vi "Lab Panel V5.22.vi"() -> ()   [LabVIEW 2013] (continued)
              n180 = call "sub vi - GET ALL TEMP v7.vi"("LA01-EN"=w224, "simulate"=w186, "LA02-EN"=w224, "LA03-EN"=w224, "LA04-EN"=w224, "LA05-EN"=w224, "Gen Cal Value"=1) -> ("LA01 TEMP"=w222:T24, "LA02 TEMP"=w215:T24, "LA03 TEMP"=w208:T24, "LA04 TEMP"=w201:T24, "LA05 TEMP"=w194:T24)  [unwired: 3 in, 1 out]
              n181 = local write "LAB05 TEMP"(w194) -> ()
              n182 = local write "LAB04 TEMP"(w201) -> ()
              n183 = Unbundle(w208) -> ("T1"=w205:dbl, "T2"=w204:dbl, "T3"=w203:dbl, "T4"=w202:dbl)  [unwired: 2 out]
              n184 = Unbundle(w222) -> ("T1"=w220:dbl, "T2"=w219:dbl, "T3"=w218:dbl, "T4"=w217:dbl)  [unwired: 2 out]
              n185 = Unbundle(w215) -> ("T1"=w212:dbl, "T2"=w211:dbl, "T3"=w210:dbl, "T4"=w209:dbl)  [unwired: 2 out]
              n186 = Unbundle(w201) -> ("T1"=w199:dbl, "T2"=w198:dbl, "T3"=w197:dbl, "T4"=w196:dbl)  [unwired: 2 out]
              n187 = Unbundle(w194) -> ("T1"=w192:dbl, "T2"=w191:dbl, "T3"=w190:dbl, "T4"=w189:dbl)  [unwired: 2 out]
              n188 = local write "LAB01 TEMP"(w222) -> ()
              n189 = local write "LAB02 TEMP"(w215) -> ()
              n190 = local write "LAB03 TEMP"(w208) -> ()
              n191 = local read "TEMP LA05"() -> (w193:T9)
              n192 = local read "TEMP LA04"() -> (w200:T9)
              n193 = local read "TEMP LA02"() -> (w214:T9)
              n194 = local read "TEMP LA03"() -> (w207:T9)
              n195 = local read "TEMP LA01"() -> (w221:T9)
              n196 = Bundle(cluster=w207, "TL-1"=w205, "TN-1"=w204, "TL-2"=w203, "TN-2"=w202) -> (w206:T9)  [unwired: 4 in]
              n197 = Bundle(cluster=w221, "TL-1"=w220, "TN-1"=w219, "TL-2"=w218, "TN-2"=w217) -> (w216:T9)  [unwired: 4 in]
              n198 = Bundle(cluster=w214, "TL-1"=w212, "TN-1"=w211, "TL-2"=w210, "TN-2"=w209) -> (w213:T9)  [unwired: 4 in]
              n199 = Bundle(cluster=w200, "TL-1"=w199, "TN-1"=w198, "TL-2"=w197, "TN-2"=w196) -> (w195:T9)  [unwired: 4 in]
              n200 = Bundle(cluster=w193, "TL-1"=w192, "TN-1"=w191, "TL-2"=w190, "TN-2"=w189) -> (w188:T9)  [unwired: 4 in]
              n201 = local write "TEMP LA03"(w206) -> ()
              n202 = local write "TEMP LA01"(w216) -> ()
              n203 = local write "TEMP LA02"(w213) -> ()
              n204 = local write "TEMP LA05"(w188) -> ()
              n205 = local write "TEMP LA04"(w195) -> ()
            }
            frame #2 {
              w235 = 0
              n206 = local read "LAB01 TEMP"() -> (w237:T12)
              n207 = local read "SIG LAB01-2"() -> (w232:T2)
              n208 = Unbundle By Name(w237) -> ("T1 Live"=w230:dbl, "T1 Neut"=w229:dbl, "T2 Live"=w228:dbl, "T2 Neut"=w227:dbl)  [unwired: 2 out]
              n209 = local read "SIG LAB01-1"() -> (w234:T2)
              n210 = local read "TEMP LA01"() -> (w238:T9)
              n211 = Bundle By Name(cluster=w238, "TL-1"=w230, "TN-1"=w229, "TL-2"=w228, "TN-2"=w227, "TL -1COUNT"=w235, "TN-1 COUNT"=w235, "TL-2 COUNT"=w235, "TN-2 COUNT"=w235) -> (w236:T9)
              n212 = Bundle(cluster=w234, "Tmp Live"=w230, "Tmp Neut"=w229) -> (w233:T2)  [unwired: 3 in]
              n213 = Bundle(cluster=w232, "Tmp Live"=w228, "Tmp Neut"=w227) -> (w231:T2)  [unwired: 3 in]
              n214 = local write "SIG LAB01-2"(w231) -> ()
              n215 = local write "SIG LAB01-1"(w233) -> ()
              n216 = local write "TEMP LA01"(w236) -> ()
            }
            frame #3 {
              w247 = 0
              n217 = local read "LAB02 TEMP"() -> (w249:T12)
              n218 = Unbundle By Name(w249) -> ("T1 Live"=w242:dbl, "T1 Neut"=w241:dbl, "T2 Live"=w240:dbl, "T2 Neut"=w239:dbl)  [unwired: 2 out]
              n219 = local read "SIG LAB02-1"() -> (w246:T2)
              n220 = local read "SIG LAB02-2"() -> (w245:T2)
              n221 = local read "TEMP LA02"() -> (w250:T9)
              n222 = Bundle By Name(cluster=w250, "TL-1"=w242, "TN-1"=w241, "TL-2"=w240, "TN-2"=w239, "TL -1COUNT"=w247, "TN-1 COUNT"=w247, "TL-2 COUNT"=w247, "TN-2 COUNT"=w247) -> (w248:T9)
              n223 = Bundle(cluster=w245, "Tmp Live"=w240, "Tmp Neut"=w239) -> (w243:T2)  [unwired: 3 in]
              n224 = Bundle(cluster=w246, "Tmp Live"=w242, "Tmp Neut"=w241) -> (w244:T2)  [unwired: 3 in]
              n225 = local write "TEMP LA02"(w248) -> ()
              n226 = local write "SIG LAB02-1"(w244) -> ()
              n227 = local write "SIG LAB02-2"(w243) -> ()
            }
            frame #4 {
              w259 = 0
              n228 = local read "LAB03 TEMP"() -> (w261:T12)
              n229 = Unbundle By Name(w261) -> ("T1 Live"=w254:dbl, "T1 Neut"=w253:dbl, "T2 Live"=w252:dbl, "T2 Neut"=w251:dbl)  [unwired: 2 out]
              n230 = local read "SIG LAB03-1"() -> (w258:T2)
              n231 = local read "SIG LAB03-2"() -> (w257:T2)
              n232 = local read "TEMP LA03"() -> (w262:T9)
              n233 = Bundle By Name(cluster=w262, "TL-1"=w254, "TN-1"=w253, "TL-2"=w252, "TN-2"=w251, "TL -1COUNT"=w259, "TN-1 COUNT"=w259, "TL-2 COUNT"=w259, "TN-2 COUNT"=w259) -> (w260:T9)
              n234 = Bundle(cluster=w257, "Tmp Live"=w252, "Tmp Neut"=w251) -> (w255:T2)  [unwired: 3 in]
              n235 = Bundle(cluster=w258, "Tmp Live"=w254, "Tmp Neut"=w253) -> (w256:T2)  [unwired: 3 in]
              n236 = local write "TEMP LA03"(w260) -> ()
              n237 = local write "SIG LAB03-2"(w255) -> ()
              n238 = local write "SIG LAB03-1"(w256) -> ()
            }
            frame #5 {
              w271 = 0
              n239 = local read "LAB04 TEMP"() -> (w273:T12)
              n240 = Unbundle By Name(w273) -> ("T1 Live"=w266:dbl, "T1 Neut"=w265:dbl, "T2 Live"=w264:dbl, "T2 Neut"=w263:dbl)  [unwired: 2 out]
              n241 = local read "SIG LAB04-2"() -> (w269:T2)
              n242 = local read "SIG LAB04-1"() -> (w270:T2)
              n243 = local read "TEMP LA04"() -> (w274:T9)
              n244 = Bundle By Name(cluster=w274, "TL-1"=w266, "TN-1"=w265, "TL-2"=w264, "TN-2"=w263, "TL -1COUNT"=w271, "TN-1 COUNT"=w271, "TL-2 COUNT"=w271, "TN-2 COUNT"=w271) -> (w272:T9)
              n245 = Bundle(cluster=w269, "Tmp Live"=w264, "Tmp Neut"=w263) -> (w267:T2)  [unwired: 3 in]
              n246 = Bundle(cluster=w270, "Tmp Live"=w266, "Tmp Neut"=w265) -> (w268:T2)  [unwired: 3 in]
              n247 = local write "SIG LAB04-2"(w267) -> ()
              n248 = local write "TEMP LA04"(w272) -> ()
              n249 = local write "SIG LAB04-1"(w268) -> ()
            }
            frame #6 {
              w283 = 0
              n250 = local read "LAB05 TEMP"() -> (w285:T12)
              n251 = Unbundle By Name(w285) -> ("T1 Live"=w278:dbl, "T1 Neut"=w277:dbl, "T2 Live"=w276:dbl, "T2 Neut"=w275:dbl)  [unwired: 2 out]
              n252 = local read "SIG LAB05-2"() -> (w281:T2)
              n253 = local read "SIG LAB05-1"() -> (w282:T2)
              n254 = local read "TEMP LA05"() -> (w286:T9)
              n255 = Bundle By Name(cluster=w286, "TL-1"=w278, "TN-1"=w277, "TL-2"=w276, "TN-2"=w275, "TL -1COUNT"=w283, "TN-1 COUNT"=w283, "TL-2 COUNT"=w283, "TN-2 COUNT"=w283) -> (w284:T9)
              n256 = Bundle(cluster=w281, "Tmp Live"=w276, "Tmp Neut"=w275) -> (w279:T2)  [unwired: 3 in]
              n257 = Bundle(cluster=w282, "Tmp Live"=w278, "Tmp Neut"=w277) -> (w280:T2)  [unwired: 3 in]
              n258 = local write "SIG LAB05-2"(w279) -> ()
              n259 = local write "SIG LAB05-1"(w280) -> ()
              n260 = local write "TEMP LA05"(w284) -> ()
            }
          }
        }
        frame #8 {
          # "enable front panel, all settings done"
          n261 = property on="Tab Control 2" class="TabCtl (strict)"("DisabledEnum"=T16."Enabled" ("Disabled")) -> ()  [unwired: 2 in, 2 out]
          n262 = property on="Tab Control 2" class="TabCtl (strict)"("Value"=0) -> ()  [unwired: 2 in, 2 out]
        }
        frame #9 {
          n263 = property on="Tab Control 2" class="TabCtl (strict)"("Value"=0) -> ()  [unwired: 2 in, 2 out]
        }
      }
    }
    frame #2 {
      n264 = node-c288("loop  delay(mS)") -> (w292:T17)  [unwired: 3 in]
      n265 = timed-loop {
        timing: w292 -> [_]
        timing-out: [_] -> w291
        i -> [w318]
        stop <- w294 stop-if-true
        n266 = node-c288() -> ()  [unwired: 1 in, 1 out]
        n267 = local read "Resets Done"() -> (w297:dbl)
        n268 = Greater?(x=w297, y=10) -> (0:w293:bool)
        n269 = local read "SELECT LAB05-2"() -> (w298:T3)
        n270 = local read "SELECT LAB05-1"() -> (w299:T3)
        n271 = local read "SELECT LAB04-2"() -> (w300:T3)
        n272 = local read "SELECT LAB03-1"() -> (w303:T3)
        n273 = local read "SELECT LAB02-2"() -> (w304:T3)
        n274 = local read "SELECT LAB01-1"() -> (w307:T3)
        n275 = local read "SELECT LAB03-2"() -> (w302:T3)
        n276 = local read "SELECT LAB01-2"() -> (w306:T3)
        n277 = local read "SELECT LAB04-1"() -> (w301:T3)
        n278 = Or(x=w293, y="stop") -> (x .or. y?=w294:bool)
        n279 = local read "SELECT LAB02-1"() -> (w305:T3)
        n280 = local read "run lab03-2"() -> (w312:bool)
        n281 = local read "run lab04-1"() -> (w311:bool)
        n282 = local read "run lab05-1"() -> (w309:bool)
        n283 = local read "run lab04-2"() -> (w310:bool)
        n284 = local read "run lab05-2"() -> (w308:bool)
        n285 = local read "run lab03-1"() -> (w313:bool)
        n286 = local read "run lab02-2"() -> (w314:bool)
        n287 = local read "run lab02-1"() -> (w315:bool)
        n288 = local read "run lab01-1"() -> (w317:bool)
        n289 = local read "run lab01-2"() -> (w316:bool)
        n290 = global write "Global display 1.vi" "stop disp"(w294) -> ()
        n291 = stacked-sequence {
          seq-local: [_ w384 _ _ _ _ _ _ _ _ _ _ _ _ _ _ _ _ _ _ _ _ _] -> [_ _ _ _ _ w2485 _ _ _ _ _ _ _ _ _ _ _ _ _ _ _ _ _]
          seq-local: [_ w383 _ _ _ _ _ _ _ _ _ _ _ _ _ _ _ _ _ _ _ _ _] -> [_ _ _ _ _ w2484 _ _ _ _ _ _ _ _ _ _ _ _ _ _ _ _ _]
          seq-local: [_ w370 _ _ _ _ _ _ _ _ _ _ _ _ _ _ _ _ _ _ _ _ _] -> [_ _ _ _ _ w2483 _ _ _ _ _ _ _ _ _ _ _ _ _ _ _ _ _]
          seq-local: [_ w369 _ _ _ _ _ _ _ _ _ _ _ _ _ _ _ _ _ _ _ _ _] -> [_ _ _ _ _ w2482 _ _ _ _ _ _ _ _ _ _ _ _ _ _ _ _ _]
          seq-local: [_ w368 _ _ _ _ _ _ _ _ _ _ _ _ _ _ _ _ _ _ _ _ _] -> [_ _ _ _ _ w2481 _ _ _ _ _ _ _ _ _ _ _ _ _ _ _ _ _]
          seq-local: [_ w367 _ _ _ _ _ _ _ _ _ _ _ _ _ _ _ _ _ _ _ _ _] -> [_ _ _ _ _ w2480 _ _ _ _ _ _ _ _ _ _ _ _ _ _ _ _ _]
          seq-local: [_ w366 _ _ _ _ _ _ _ _ _ _ _ _ _ _ _ _ _ _ _ _ _] -> [_ _ _ _ _ w2479 _ _ _ _ _ _ _ _ _ _ _ _ _ _ _ _ _]
          seq-local: [_ w365 _ _ _ _ _ _ _ _ _ _ _ _ _ _ _ _ _ _ _ _ _] -> [_ _ _ _ _ w2478 _ _ _ _ _ _ _ _ _ _ _ _ _ _ _ _ _]
          seq-local: [_ w364 _ _ _ _ _ _ _ _ _ _ _ _ _ _ _ _ _ _ _ _ _] -> [_ _ _ _ _ w2477 _ _ _ _ _ _ _ _ _ _ _ _ _ _ _ _ _]
          seq-local: [_ w363 _ _ _ _ _ _ _ _ _ _ _ _ _ _ _ _ _ _ _ _ _] -> [_ _ _ _ _ w2476 _ _ _ _ _ _ _ _ _ _ _ _ _ _ _ _ _]
          tunnel: w317 -> [_ _ w400 w648 w2075 w2505 w2820 w3307 _ _ _ _ w3867 _ w4824 _ _ w5112 w5415 w5597 _ _ _]
          tunnel: w316 -> [_ _ w399 w646 w2074 w2504 w2821 w3306 _ _ _ _ w3866 _ w4822 _ _ w5111 w5414 w5595 _ _ _]
          tunnel: w315 -> [_ _ w398 w644 w2073 w2503 w2819 w3305 _ _ _ _ w3865 _ w4820 _ _ w5110 w5413 w5594 _ _ _]
          tunnel: w314 -> [_ _ w397 w642 w2072 w2502 w2818 w3304 _ _ _ _ w3864 _ w4818 _ _ w5109 w5412 w5593 _ _ _]
          tunnel: w313 -> [_ _ w396 w640 w2071 w2501 w2817 w3303 _ _ _ _ w3863 _ w4816 _ _ w5108 w5411 w5592 _ _ _]
          tunnel: w312 -> [_ _ w395 w638 w2070 w2500 w2816 w3302 _ _ _ _ w3862 _ w4814 _ _ w5107 w5410 w5591 _ _ _]
          tunnel: w311 -> [_ _ w394 w636 w2069 w2499 w2815 w3301 _ _ _ _ w3861 _ w4812 _ _ w5106 w5409 w5590 _ _ _]
          tunnel: w310 -> [_ _ w393 w634 w2068 w2498 w2814 w3300 _ _ _ _ w3860 _ w4810 _ _ w5105 w5408 w5589 _ _ _]
          tunnel: w309 -> [_ _ w392 w632 w2067 w2497 w2813 w3299 _ _ _ _ w3859 _ w4808 _ _ w5104 w5407 w5588 _ _ _]
          tunnel: w308 -> [_ _ w391 w630 w2066 w2496 w2812 w3298 _ _ _ _ w3858 _ w4806 _ _ w5103 w5406 w5587 _ _ _]
          tunnel: w307 -> [_ _ _ w647 w2065 w2495 _ _ _ _ _ _ _ _ w4826 _ _ _ _ _ w5942 _ _]
          tunnel: w306 -> [_ _ _ w645 w2064 w2494 _ _ _ _ _ _ _ _ w4821 _ _ _ _ _ w5941 _ _]
          tunnel: w305 -> [_ _ _ w643 w2063 w2493 _ _ _ _ _ _ _ _ w4819 _ _ _ _ _ w5940 _ _]
          tunnel: w304 -> [_ _ _ w641 w2062 w2492 _ _ _ _ _ _ _ _ w4817 _ _ _ _ _ w5939 _ _]
          tunnel: w303 -> [_ _ _ w639 w2061 w2491 _ _ _ _ _ _ _ _ w4815 _ _ _ _ _ w5938 _ _]
          tunnel: w302 -> [_ _ _ w637 w2060 w2490 _ _ _ _ _ _ _ _ w4813 _ _ _ _ _ w5937 _ _]
          tunnel: w301 -> [_ _ _ w635 w2059 w2489 _ _ _ _ _ _ _ _ w4811 _ _ _ _ _ w5936 _ _]
          tunnel: w300 -> [_ _ _ w633 w2058 w2488 _ _ _ _ _ _ _ _ w4809 _ _ _ _ _ w5935 _ _]
          tunnel: w299 -> [_ _ _ w631 w2057 w2487 _ _ _ _ _ _ _ _ w4807 _ _ _ _ _ w5934 _ _]
          tunnel: w298 -> [_ _ _ w629 w2056 w2486 _ _ _ _ _ _ _ _ w4805 _ _ _ _ _ w5933 _ _]
          tunnel: w293 -> [_ _ _ _ _ _ _ _ _ _ _ _ _ _ _ _ _ _ _ _ _ _ w5994]
          frame #0 {
            w326 = FALSE
            w331 = 0.5
            # "set up cycle control"
            n292 = local read "jig cycle"() -> (w330:dbl)
            n293 = local read "Amps Fail level"() -> (w324:dbl)
            n294 = local read "Simulate"() -> (w321:bool)
            n295 = Divide(x="JIG ON TIME (S)", y=w331) -> (x/y=→"on loops":dbl)
            n296 = Divide(x="JIG OFF TIME (S)", y=w331) -> (x/y=→"off loops":dbl)
            n297 = Increment(x=w330) -> (x+1=w329:dbl)
            n298 = local write "Simulate IND"(w321) -> ()
            n299 = global write "Global display 3.vi" "Amps Fail"(w324) -> ()
            n300 = local write "TEMP"(w326) -> ()
            n301 = local write "AI"(w326) -> ()
            n302 = local read "Network Directory"() -> (w323:path)
            n303 = local write "jig cycle"(w329) -> ()
            n304 = call "sub vi - check network dir v2.vi"("PATH"=w323) -> ("error"=w322:bool)  [unwired: 10 in]
            n305 = local write "network error"(w322) -> ()
            n306 = global write "Global display 3.vi" "network drive"(w322) -> ()
            n307 = event shown="[1] \"ADMIN\": Value Change" {
              selector: _ -> [_ _]
              dyn-events: _ -> [_ _]
              timeout: 10 -> [_ _]
              event Timeout {
                n308 = event-data() -> ()  [unwired: 1 in, 3 out]
              }
              event "ADMIN": Value Change {
                n309 = event-data() -> ()  [unwired: 1 in, 6 out]
                n310 = stacked-sequence {
                  seq-local: [_ w335 _] -> [_ _ w336]
                  frame #0 {
                    n311 = global write "Global 1.vi" "password"("9949") -> ()
                  }
                  frame #1 {
                    n312 = call "sub vi - password 1.vi"() -> ("RESULT"=w335:bool)  [unwired: 11 in]
                  }
                  frame #2 {
                    w338 = FALSE
                    n313 = property on="Tab Control 2" class="TabCtl (strict)"() -> ("Pages"=w342:refnum<vi>[])  [unwired: 2 in, 2 out]
                    n314 = Select(t=TRUE, s=w336, f=w338) -> (s? t:f=w337:bool)
                    n315 = Index Array(array=w342, index=8) -> (element=w340:refnum<vi>)
                    n316 = property class="Page"(reference=w340, "PageVis"=w337) -> ()  [unwired: 1 in, 2 out]
                    n317 = local write "ADMIN"(w338) -> ()
                  }
                }
              }
            }
          }
          frame #1 {
            w380 = 60.0
            # "convert temperature rise minutes to cycles"
            n318 = local read "SET LAB05-2"() -> (w344:T5)
            n319 = local read "SET LAB05-1"() -> (w346:T5)
            n320 = local read "SET LAB04-2"() -> (w348:T5)
            n321 = local read "SET LAB01-1"() -> (w362:T5)
            n322 = local read "SET LAB01-2"() -> (w360:T5)
            n323 = local read "SET LAB02-2"() -> (w356:T5)
            n324 = local read "SET LAB04-1"() -> (w350:T5)
            n325 = local read "SET LAB03-1"() -> (w354:T5)
            n326 = local read "SET LAB03-2"() -> (w352:T5)
            n327 = local read "SET LAB02-1"() -> (w358:T5)
            n328 = local read "JIG OFF TIME (S)"() -> (w385:dbl)
            n329 = local read "JIG ON TIME (S)"() -> (w386:dbl)
            n330 = Unbundle(w344) -> ("T-RISE mins"=w343:dbl)  [unwired: 4 out]
            n331 = Unbundle(w346) -> ("T-RISE mins"=w345:dbl)  [unwired: 4 out]
            n332 = Unbundle(w362) -> ("T-RISE mins"=w361:dbl)  [unwired: 4 out]
            n333 = Unbundle(w348) -> ("T-RISE mins"=w347:dbl)  [unwired: 4 out]
            n334 = Unbundle(w360) -> ("T-RISE mins"=w359:dbl)  [unwired: 4 out]
            n335 = Unbundle(w358) -> ("T-RISE mins"=w357:dbl)  [unwired: 4 out]
            n336 = Unbundle(w350) -> ("T-RISE mins"=w349:dbl)  [unwired: 4 out]
            n337 = Unbundle(w356) -> ("T-RISE mins"=w355:dbl)  [unwired: 4 out]
            n338 = Unbundle(w352) -> ("T-RISE mins"=w351:dbl)  [unwired: 4 out]
            n339 = Unbundle(w354) -> ("T-RISE mins"=w353:dbl)  [unwired: 4 out]
            n340 = Add(x=w386, y=w385) -> (x+y=w379:dbl)
            n341 = Multiply(x=w380, y=w351) -> (x*y=w375:dbl)
            n342 = Multiply(x=w380, y=w349) -> (x*y=w374:dbl)
            n343 = Multiply(x=w380, y=w347) -> (x*y=w373:dbl)
            n344 = Multiply(x=w380, y=w345) -> (x*y=w372:dbl)
            n345 = Multiply(x=w380, y=w343) -> (x*y=w371:dbl)
            n346 = Multiply(x=w380, y=w359) -> (x*y=w381:dbl)
            n347 = Multiply(x=w380, y=w353) -> (x*y=w376:dbl)
            n348 = Multiply(x=w380, y=w361) -> (x*y=w382:dbl)
            n349 = Multiply(x=w380, y=w357) -> (x*y=w378:dbl)
            n350 = Multiply(x=w380, y=w355) -> (x*y=w377:dbl)
            n351 = Divide(x=w372, y=w379) -> (x/y=w364:dbl)
            n352 = Divide(x=w373, y=w379) -> (x/y=w365:dbl)
            n353 = Divide(x=w374, y=w379) -> (x/y=w366:dbl)
            n354 = Divide(x=w371, y=w379) -> (x/y=w363:dbl)
            n355 = Divide(x=w376, y=w379) -> (x/y=w368:dbl)
            n356 = Divide(x=w382, y=w379) -> (x/y=w384:dbl)
            n357 = Divide(x=w381, y=w379) -> (x/y=w383:dbl)
            n358 = Divide(x=w378, y=w379) -> (x/y=w370:dbl)
            n359 = Divide(x=w377, y=w379) -> (x/y=w369:dbl)
            n360 = Divide(x=w375, y=w379) -> (x/y=w367:dbl)
          }
          frame #2 {
            # "control cycle loops"
            n361 = local read "JIG OFF TIME (S)"() -> (w389:dbl)
            n362 = local read "JIG ON TIME (S)"() -> (w388:dbl)
            n363 = local read "jig cycle"() -> (w402:dbl)
            n364 = local read "on loops"() -> (w404:dbl)
            n365 = local read "off loops"() -> (w403:dbl)
            n366 = Add(x=w389, y=w388) -> (x+y=w387:dbl)
            n367 = Add(x=w404, y=w403) -> (x+y=w390:dbl)
            n368 = Greater Or Equal?(x=w402, y=w390) -> (x >= y?=w401:bool)
            n369 = case shown="True" w401 {
              tunnel: w400 -> [_ w438]
              tunnel: w399 -> [_ w437]
              tunnel: w398 -> [_ w436]
              tunnel: w397 -> [_ w435]
              tunnel: w396 -> [_ w434]
              tunnel: w395 -> [_ w433]
              tunnel: w394 -> [_ w432]
              tunnel: w393 -> [_ w431]
              tunnel: w392 -> [_ w430]
              tunnel: w391 -> [_ w429]
              tunnel: w387 -> [_ w428]
              frame False {
              }
              frame True {
                # "increment cycle value and convert cycles to minutes for temp rise"
                n370 = stacked-sequence {
                  frame #0 {
                    n371 = local read "Panel #"() -> (w441:dbl)
                    n372 = Increment(x=w441) -> (x+1=w440:dbl)
                    n373 = local write "Panel #"(w440) -> ()
                  }
                  frame #1 {
                    n374 = local read "Panel #"() -> (w442:dbl)
                    n375 = Greater?(x=w442, y=5) -> (0:w444:bool)
                    n376 = case shown="True" w444 {
                      frame False {
                      }
                      frame True {
                        n377 = local write "Panel #"(1) -> ()
                      }
                    }
                  }
                }
                n378 = local read "JIG RELAY CYCLES"() -> (w427:T8)
                n379 = local read "Panel #"() -> (→"Tp Ut":dbl)
                n380 = Unbundle By Name(w427) -> ("LAB01-1"=w425:dbl, "LAB01-2"=w423:dbl, "LAB02-1"=w421:dbl, "LAB02-2"=w419:dbl, "LAB03-1"=w417:dbl, "LAB03-2"=w415:dbl, "LAB04-1"=w413:dbl, "LAB04-2"=w411:dbl, "LAB05-1"=w409:dbl, "LAB05-2"=w407:dbl)
                n381 = stacked-sequence {
                  tunnel: w438 -> [w456 _ _ _ _ _ _ _ _ _]
                  tunnel: w437 -> [_ w473 _ _ _ _ _ _ _ _]
                  tunnel: w436 -> [_ _ w490 _ _ _ _ _ _ _]
                  tunnel: w435 -> [_ _ _ w507 _ _ _ _ _ _]
                  tunnel: w434 -> [_ _ _ _ w524 _ _ _ _ _]
                  tunnel: w433 -> [_ _ _ _ _ w541 _ _ _ _]
                  tunnel: w432 -> [_ _ _ _ _ _ w558 _ _ _]
                  tunnel: w431 -> [_ _ _ _ _ _ _ w575 _ _]
                  tunnel: w430 -> [_ _ _ _ _ _ _ _ w592 _]
                  tunnel: w429 -> [_ _ _ _ _ _ _ _ _ w609]
                  tunnel: w428 -> [w453 w470 w487 w504 w521 w538 w555 w572 w589 w606]
                  tunnel: w425 -> [w447 _ _ _ _ _ _ _ _ _]
                  tunnel: [w446 _ _ _ _ _ _ _ _ _] -> w424
                  tunnel: w423 -> [_ w464 _ _ _ _ _ _ _ _]
                  tunnel: [_ w463 _ _ _ _ _ _ _ _] -> w422
                  tunnel: w421 -> [_ _ w481 _ _ _ _ _ _ _]
                  tunnel: [_ _ w480 _ _ _ _ _ _ _] -> w420
                  tunnel: w419 -> [_ _ _ w498 _ _ _ _ _ _]
                  tunnel: [_ _ _ w497 _ _ _ _ _ _] -> w418
                  tunnel: w417 -> [_ _ _ _ w515 _ _ _ _ _]
                  tunnel: [_ _ _ _ w514 _ _ _ _ _] -> w416
                  tunnel: w415 -> [_ _ _ _ _ w532 _ _ _ _]
                  tunnel: [_ _ _ _ _ w531 _ _ _ _] -> w414
                  tunnel: w413 -> [_ _ _ _ _ _ w549 _ _ _]
                  tunnel: [_ _ _ _ _ _ w548 _ _ _] -> w412
                  tunnel: w411 -> [_ _ _ _ _ _ _ w566 _ _]
                  tunnel: [_ _ _ _ _ _ _ w565 _ _] -> w410
                  tunnel: w409 -> [_ _ _ _ _ _ _ _ w583 _]
                  tunnel: [_ _ _ _ _ _ _ _ w582 _] -> w408
                  tunnel: w407 -> [_ _ _ _ _ _ _ _ _ w600]
                  tunnel: [_ _ _ _ _ _ _ _ _ w599] -> w406
                  frame #0 {
                    n382 = local read "DISP LAB01-1"() -> (w451:T4)
                    n383 = Unbundle(w451) -> ("CYCLE"=w452:dbl)  [unwired: 2 out]
                    n384 = case shown="True" w456 {
                      tunnel: w452 -> [w458 w462]
                      tunnel: [w458 w461] -> w450
                      tunnel: w447 -> [w457 w460]
                      tunnel: [w457 w459] -> w446
                      frame False {
                      }
                      frame True {
                        n385 = Increment(x=w460) -> (x+1=w459:dbl)
                        n386 = Increment(x=w462) -> (x+1=w461:dbl)
                      }
                    }
                    n387 = Multiply(x=w450, y=w453) -> (x*y=w454:dbl)
                    n388 = Divide(x=w454, y=60.0) -> (x/y=w449:dbl)
                    n389 = Bundle(cluster=w451, "CYCLE"=w450, "MINS"=w449) -> (w448:T4)  [unwired: 1 in]
                    n390 = local write "DISP LAB01-1"(w448) -> ()
                  }
                  frame #1 {
                    n391 = local read "DISP LAB01-2"() -> (w468:T4)
                    n392 = Unbundle(w468) -> ("CYCLE"=w469:dbl)  [unwired: 2 out]
                    n393 = case shown="True" w473 {
                      tunnel: w469 -> [w475 w479]
                      tunnel: [w475 w478] -> w466
                      tunnel: w464 -> [w474 w477]
                      tunnel: [w474 w476] -> w463
                      frame False {
                      }
                      frame True {
                        n394 = Increment(x=w477) -> (x+1=w476:dbl)
                        n395 = Increment(x=w479) -> (x+1=w478:dbl)
                      }
                    }
                    n396 = Multiply(x=w466, y=w470) -> (x*y=w471:dbl)
                    n397 = Divide(x=w471, y=60.0) -> (x/y=w465:dbl)
                    n398 = Bundle(cluster=w468, "CYCLE"=w466, "MINS"=w465) -> (w467:T4)  [unwired: 1 in]
                    n399 = local write "DISP LAB01-2"(w467) -> ()
                  }
                  frame #2 {
                    n400 = local read "DISP LAB02-1"() -> (w485:T4)
                    n401 = Unbundle(w485) -> ("CYCLE"=w486:dbl)  [unwired: 2 out]
                    n402 = case shown="True" w490 {
                      tunnel: [w492 w496] -> w483
                      tunnel: w486 -> [w492 w495]
                      tunnel: w481 -> [w491 w494]
                      tunnel: [w491 w493] -> w480
                      frame False {
                      }
                      frame True {
                        n403 = Increment(x=w494) -> (x+1=w493:dbl)
                        n404 = Increment(x=w495) -> (x+1=w496:dbl)
                      }
                    }
                    n405 = Multiply(x=w483, y=w487) -> (x*y=w488:dbl)
                    n406 = Divide(x=w488, y=60.0) -> (x/y=w482:dbl)
                    n407 = Bundle(cluster=w485, "CYCLE"=w483, "MINS"=w482) -> (w484:T4)  [unwired: 1 in]
                    n408 = local write "DISP LAB02-1"(w484) -> ()
                  }
                  frame #3 {
                    n409 = local read "DISP LAB02-2"() -> (w502:T4)
                    n410 = Unbundle(w502) -> ("CYCLE"=w503:dbl)  [unwired: 2 out]
                    n411 = case shown="True" w507 {
                      tunnel: [w509 w513] -> w501
                      tunnel: w503 -> [w509 w512]
                      tunnel: w498 -> [w508 w511]
                      tunnel: [w508 w510] -> w497
                      frame False {
                      }
                      frame True {
                        n412 = Increment(x=w511) -> (x+1=w510:dbl)
                        n413 = Increment(x=w512) -> (x+1=w513:dbl)
                      }
                    }
                    n414 = Multiply(x=w501, y=w504) -> (x*y=w505:dbl)
                    n415 = Divide(x=w505, y=60.0) -> (x/y=w500:dbl)
                    n416 = Bundle(cluster=w502, "CYCLE"=w501, "MINS"=w500) -> (w499:T4)  [unwired: 1 in]
                    n417 = local write "DISP LAB02-2"(w499) -> ()
                  }
                  frame #4 {
                    n418 = local read "DISP LAB03-1"() -> (w519:T4)
                    n419 = Unbundle(w519) -> ("CYCLE"=w520:dbl)  [unwired: 2 out]
                    n420 = case shown="True" w524 {
                      tunnel: [w526 w530] -> w516
                      tunnel: w520 -> [w526 w529]
                      tunnel: w515 -> [w525 w528]
                      tunnel: [w525 w527] -> w514
                      frame False {
                      }
                      frame True {
                        n421 = Increment(x=w528) -> (x+1=w527:dbl)
                        n422 = Increment(x=w529) -> (x+1=w530:dbl)
                      }
                    }
                    n423 = Multiply(x=w516, y=w521) -> (x*y=w522:dbl)
                    n424 = Divide(x=w522, y=60.0) -> (x/y=w517:dbl)
                    n425 = Bundle(cluster=w519, "CYCLE"=w516, "MINS"=w517) -> (w518:T4)  [unwired: 1 in]
                    n426 = local write "DISP LAB03-1"(w518) -> ()
                  }
                  frame #5 {
                    n427 = local read "DISP LAB03-2"() -> (w536:T4)
                    n428 = Unbundle(w536) -> ("CYCLE"=w537:dbl)  [unwired: 2 out]
                    n429 = case shown="True" w541 {
                      tunnel: [w543 w547] -> w535
                      tunnel: w537 -> [w543 w546]
                      tunnel: w532 -> [w542 w545]
                      tunnel: [w542 w544] -> w531
                      frame False {
                      }
                      frame True {
                        n430 = Increment(x=w545) -> (x+1=w544:dbl)
                        n431 = Increment(x=w546) -> (x+1=w547:dbl)
                      }
                    }
                    n432 = Multiply(x=w535, y=w538) -> (x*y=w539:dbl)
                    n433 = Divide(x=w539, y=60.0) -> (x/y=w534:dbl)
                    n434 = Bundle(cluster=w536, "CYCLE"=w535, "MINS"=w534) -> (w533:T4)  [unwired: 1 in]
                    n435 = local write "DISP LAB03-2"(w533) -> ()
                  }
                  frame #6 {
                    n436 = local read "DISP LAB04-1"() -> (w553:T4)
                    n437 = Unbundle(w553) -> ("CYCLE"=w554:dbl)  [unwired: 2 out]
                    n438 = case shown="True" w558 {
                      tunnel: [w560 w564] -> w551
                      tunnel: w554 -> [w560 w563]
                      tunnel: w549 -> [w559 w562]
                      tunnel: [w559 w561] -> w548
                      frame False {
                      }
                      frame True {
                        n439 = Increment(x=w562) -> (x+1=w561:dbl)
                        n440 = Increment(x=w563) -> (x+1=w564:dbl)
                      }
                    }
                    n441 = Multiply(x=w551, y=w555) -> (x*y=w556:dbl)
                    n442 = Divide(x=w556, y=60.0) -> (x/y=w550:dbl)
                    n443 = Bundle(cluster=w553, "CYCLE"=w551, "MINS"=w550) -> (w552:T4)  [unwired: 1 in]
                    n444 = local write "DISP LAB04-1"(w552) -> ()
                  }
                  frame #7 {
                    n445 = local read "DISP LAB04-2"() -> (w570:T4)
                    n446 = Unbundle(w570) -> ("CYCLE"=w571:dbl)  [unwired: 2 out]
                    n447 = case shown="True" w575 {
                      tunnel: [w577 w581] -> w568
                      tunnel: w571 -> [w577 w580]
                      tunnel: w566 -> [w576 w579]
                      tunnel: [w576 w578] -> w565
                      frame False {
                      }
                      frame True {
                        n448 = Increment(x=w579) -> (x+1=w578:dbl)
                        n449 = Increment(x=w580) -> (x+1=w581:dbl)
                      }
                    }
                    n450 = Multiply(x=w568, y=w572) -> (x*y=w574:dbl)
                    n451 = Divide(x=w574, y=60.0) -> (x/y=w567:dbl)
                    n452 = Bundle(cluster=w570, "CYCLE"=w568, "MINS"=w567) -> (w569:T4)  [unwired: 1 in]
                    n453 = local write "DISP LAB04-2"(w569) -> ()
                  }
                  frame #8 {
                    n454 = local read "DISP LAB05-1"() -> (w587:T4)
                    n455 = Unbundle(w587) -> ("CYCLE"=w588:dbl)  [unwired: 2 out]
                    n456 = case shown="True" w592 {
                      tunnel: [w594 w598] -> w585
                      tunnel: w588 -> [w594 w597]
                      tunnel: w583 -> [w593 w596]
                      tunnel: [w593 w595] -> w582
                      frame False {
                      }
                      frame True {
                        n457 = Increment(x=w596) -> (x+1=w595:dbl)
                        n458 = Increment(x=w597) -> (x+1=w598:dbl)
                      }
                    }
                    n459 = Multiply(x=w585, y=w589) -> (x*y=w590:dbl)
                    n460 = Divide(x=w590, y=60.0) -> (x/y=w584:dbl)
                    n461 = Bundle(cluster=w587, "CYCLE"=w585, "MINS"=w584) -> (w586:T4)  [unwired: 1 in]
                    n462 = local write "DISP LAB05-1"(w586) -> ()
                  }
                  frame #9 {
                    n463 = local read "DISP LAB05-2"() -> (w605:T4)
                    n464 = Unbundle(w605) -> ("CYCLE"=w604:dbl)  [unwired: 2 out]
                    n465 = case shown="True" w609 {
                      tunnel: [w611 w615] -> w603
                      tunnel: w604 -> [w611 w614]
                      tunnel: w600 -> [w610 w613]
                      tunnel: [w610 w612] -> w599
                      frame False {
                      }
                      frame True {
                        n466 = Increment(x=w613) -> (x+1=w612:dbl)
                        n467 = Increment(x=w614) -> (x+1=w615:dbl)
                      }
                    }
                    n468 = Multiply(x=w603, y=w606) -> (x*y=w607:dbl)
                    n469 = Divide(x=w607, y=60.0) -> (x/y=w602:dbl)
                    n470 = Bundle(cluster=w605, "CYCLE"=w603, "MINS"=w602) -> (w601:T4)  [unwired: 1 in]
                    n471 = local write "DISP LAB05-2"(w601) -> ()
                  }
                }
                n472 = local write "jig cycle"(0) -> ()
                n473 = Bundle By Name(cluster=w427, "LAB01-1"=w424, "LAB01-2"=w422, "LAB02-1"=w420, "LAB02-2"=w418, "LAB03-1"=w416, "LAB03-2"=w414, "LAB04-1"=w412, "LAB04-2"=w410, "LAB05-1"=w408, "LAB05-2"=w406) -> (w426:T8)
                n474 = local write "JIG RELAY CYCLES"(w426) -> ()
              }
            }
          }
          frame #3 {
            # "START & STOP test RUN switch change, start test if true and stop test if false"
            n475 = Get Date/Time In Seconds() -> (seconds since 1Jan1904=w627:timestamp)
            n476 = local read "C drive data root dir"() -> (w620:path)
            n477 = Format Date/Time String(time format string (%c)="%b\\%a%d", seconds (now)=w627) -> (date/time string=w651:string)  [unwired: 1 in]
            n478 = Format Date/Time String(time format string (%c)="%H%M", seconds (now)=w627) -> (date/time string=w649:string)  [unwired: 1 in]
            n479 = Format Date/Time String(time format string (%c)="LabPanel%Y", seconds (now)=w627) -> (date/time string=w626:string)  [unwired: 1 in]
            n480 = Path To String(path=w620) -> (string=w623:string)
            n481 = global write "Global 1.vi" "C drive root path"(w620) -> ()
            n482 = local read "Ref deg C"() -> (w616:dbl)
            n483 = Concatenate Strings(w623, "\\") -> (w621:string)
            n484 = event shown="[1] \"RUN LAB01-1\": Value Change" {
              selector: _ -> [_ _ _ _ _ _ _ _ _ _ _]
              dyn-events: _ -> [_ _ _ _ _ _ _ _ _ _ _]
              timeout: 10 -> [_ _ _ _ _ _ _ _ _ _ _]
              tunnel: w621 -> [_ w664 w804 w945 w1085 w1225 w1365 w1505 w1645 w1785 w1926]
              tunnel: w651 -> [_ w663 w803 w944 w1084 w1224 w1364 w1504 w1644 w1784 w1925]
              tunnel: w649 -> [_ w661 w802 w943 w1083 w1223 w1363 w1503 w1643 w1783 w1924]
              tunnel: w647 -> [_ w662 _ _ _ _ _ _ _ _ _]
              tunnel: w648 -> [_ _ _ _ _ _ _ _ _ _ _]
              tunnel: w646 -> [_ _ _ _ _ _ _ _ _ _ _]
              tunnel: w645 -> [_ _ w801 _ _ _ _ _ _ _ _]
              tunnel: w644 -> [_ _ _ _ _ _ _ _ _ _ _]
              tunnel: w643 -> [_ _ _ w942 _ _ _ _ _ _ _]
              tunnel: w642 -> [_ _ _ _ _ _ _ _ _ _ _]
              tunnel: w641 -> [_ _ _ _ w1082 _ _ _ _ _ _]
              tunnel: w640 -> [_ _ _ _ _ _ _ _ _ _ _]
              tunnel: w639 -> [_ _ _ _ _ w1222 _ _ _ _ _]
              tunnel: w638 -> [_ _ _ _ _ _ _ _ _ _ _]
              tunnel: w637 -> [_ _ _ _ _ _ w1362 _ _ _ _]
              tunnel: w636 -> [_ _ _ _ _ _ _ _ _ _ _]
              tunnel: w635 -> [_ _ _ _ _ _ _ w1502 _ _ _]
              tunnel: w634 -> [_ _ _ _ _ _ _ _ _ _ _]
              tunnel: w633 -> [_ _ _ _ _ _ _ _ w1642 _ _]
              tunnel: w632 -> [_ _ _ _ _ _ _ _ _ _ _]
              tunnel: w631 -> [_ _ _ _ _ _ _ _ _ w1782 _]
              tunnel: w630 -> [_ _ _ _ _ _ _ _ _ _ _]
              tunnel: w629 -> [_ _ _ _ _ _ _ _ _ _ w1923]
              tunnel: w626 -> [_ w660 w800 w941 w1081 w1221 w1361 w1501 w1641 w1781 w1922]
              tunnel: [_ w659 w799 w940 w1080 w1220 w1360 w1500 w1640 w1780 w1921] -> w624
              tunnel: "RESET CYCLES TO ZERO?" -> [_ w658 w797 w938 w1078 w1218 w1358 w1498 w1638 w1778 w1919]
              tunnel: "YES" -> [_ w657 w796 w937 w1077 w1217 w1357 w1497 w1637 w1777 w1918]
              tunnel: "NO" -> [_ w656 w795 w936 w1076 w1216 w1356 w1496 w1636 w1776 w1917]
              tunnel: w616 -> [_ w653 w794 w934 w1075 w1215 w1355 w1495 w1635 w1775 w1915]
              event Timeout {
                n485 = event-data() -> ()  [unwired: 1 in, 3 out]
              }
              event "RUN LAB01-1": Value Change {
                n486 = event-data() -> ("NewVal"=w654:bool)  [unwired: 1 in, 5 out]
                n487 = local read "SIG LAB01-1"() -> (w655:T2)
                n488 = local write "run lab01-1"(w654) -> ()
                n489 = case shown="True" w654 {
                  tunnel: w664 -> [_ w702]
                  tunnel: w663 -> [_ w701]
                  tunnel: w662 -> [w666 w700]
                  tunnel: w661 -> [_ w699]
                  tunnel: w660 -> [_ w698]
                  tunnel: [w665 w697] -> w659
                  tunnel: w658 -> [_ w696]
                  tunnel: w657 -> [_ w695]
                  tunnel: w656 -> [_ w694]
                  tunnel: w655 -> [_ w693]
                  tunnel: w653 -> [_ w692]
                  frame False {
                    # "stop test"
                    n490 = stacked-sequence {
                      tunnel: w666 -> [_ w678 _]
                      tunnel: [_ w670 _] -> w665
                      frame #0 {
                        n491 = local read "DISP LAB01-1"() -> (w669:T4)
                        n492 = Bundle(cluster=w669, "STATUS"="STOP") -> (w667:T4)  [unwired: 2 in]
                        n493 = local write "DISP LAB01-1"(w667) -> ()
                      }
                      frame #1 {
                        n494 = local read "DISP LAB01-1"() -> (w677:T4)
                        n495 = Unbundle(w677) -> ("CYCLE"=w675:dbl, "MINS"=w676:dbl)  [unwired: 1 out]
                        n496 = case shown="\"CYCLE TEST\"" w678 {
                          tunnel: w676 -> [_ _ w685]
                          tunnel: w675 -> [w683 w684 _]
                          tunnel: [w683 w684 w685] -> w674
                          frame "CHART TEST", Default {
                          }
                          frame "CYCLE TEST" {
                          }
                          frame "T-RISE TEST" {
                          }
                        }
                        n497 = local read "TDMS LAB01-1"() -> (w682:refnum<k34>)
                        n498 = Build Array("STOPPED") -> (w679:string[])
                        n499 = Build Array(w674) -> (w673:dbl[])
                        n500 = TDMS Write(0:w682, 5:"TEST RESULT", 7:w679, 9:w673) -> (4:w671:refnum<k34>, 15:w672:errorcluster)  [unwired: 2 in, 2 out]
                        n501 = TDMS Close(8:w672, 11:w671) -> (0:w670:errorcluster)  [unwired: 1 out]
                      }
                      frame #2 {
                        n502 = stacked-sequence {
                          tunnel: "LAB01-1" -> [w688 w690]
                          frame #0 {
                            n503 = call "sub vi - defrag tdms v1.vi"("panel id"=w688) -> ("error out"=w687:errorcluster)  [unwired: 10 in]
                            n504 = local write "data file error"(w687) -> ()
                          }
                          frame #1 {
                            n505 = call "Save data file (stop) v3.vi"("panel id"=w690) -> ("network file save error"=w689:errorcluster)  [unwired: 9 in, 1 out]
                            n506 = local write "RESULT LAB01-1"(FALSE) -> ()
                            n507 = local write "data file error"(w689) -> ()
                          }
                        }
                      }
                    }
                  }
                  frame True {
                    n508 = stacked-sequence {
                      seq-local: [w704 _] -> [_ w708]
                      tunnel: w702 -> [_ w718]
                      tunnel: w701 -> [_ w717]
                      tunnel: w700 -> [_ w716]
                      tunnel: w699 -> [_ w715]
                      tunnel: w698 -> [_ w714]
                      tunnel: [_ w713] -> w697
                      tunnel: w696 -> [_ w712]
                      tunnel: w695 -> [_ w711]
                      tunnel: w694 -> [_ w710]
                      tunnel: w693 -> [w706 w709]
                      tunnel: w692 -> [_ w707]
                      frame #0 {
                        n509 = Unbundle(w706) -> ("AMPS"=w705:dbl)  [unwired: 4 out]
                        n510 = call "Check For Amps on v1.vi"("ID"="LAB01-1", "amps"=w705) -> ("amps"=w704:bool)  [unwired: 9 in]
                      }
                      frame #1 {
                        n511 = case shown="True" w708 {
                          tunnel: w718 -> [_ w731]
                          tunnel: w717 -> [_ w730]
                          tunnel: w716 -> [_ w729]
                          tunnel: w715 -> [_ w728]
                          tunnel: w714 -> [_ w727]
                          tunnel: [errorcluster {"status"=FALSE, "code"=0, "source"=""} ("error out") w726] -> w713
                          tunnel: w712 -> [_ w725]
                          tunnel: w711 -> [_ w724]
                          tunnel: w710 -> [_ w723]
                          tunnel: w709 -> [_ w722]
                          tunnel: w707 -> [_ w721]
                          frame False {
                            w719 = FALSE
                            n512 = local write "RUN LAB01-1"(w719) -> ()
                            n513 = local write "run lab01-1"(w719) -> ()
                          }
                          frame True {
                            n514 = stacked-sequence {
                              seq-local: [w732 _ _ _ _] -> [_ w753 _ _ _]
                              tunnel: w731 -> [w737 _ _ _ _]
                              tunnel: w730 -> [w733 _ _ _ _]
                              tunnel: w729 -> [w747 _ _ _ _]
                              tunnel: w728 -> [w740 _ _ _ _]
                              tunnel: w727 -> [w735 _ _ _ _]
                              tunnel: [_ w754 _ _ _] -> w726
                              tunnel: w725 -> [_ _ _ w775 _]
                              tunnel: w724 -> [_ _ _ w785 _]
                              tunnel: w723 -> [_ _ _ w784 _]
                              tunnel: w722 -> [_ _ _ _ _]
                              tunnel: w721 -> [_ _ _ _ w791]
                              frame #0 {
                                w734 = "\\"
                                n515 = case shown="\"CHART TEST\", Default" w747 {
                                tunnel: ["L01-1-CHART TEST-" "L01-1-CYCLE TEST-" "L01-1-T-RISE TEST-"] -> w743
                                frame "CHART TEST", Default {
                                }
                                frame "CYCLE TEST" {
                                }
                                frame "T-RISE TEST" {
                                }
                                }
                                n516 = local read "SET LAB01-1"() -> (w742:T5)
                                n517 = Unbundle(w742) -> ("DESCRIPTION"=w741:string)  [unwired: 4 out]
                                n518 = Concatenate Strings(w737, "\\", w735, w734, w733, w734) -> (w744:string)
                                n519 = String To Path(string=w744) -> (path=w746:path)
                                n520 = Concatenate Strings(w744, w743, w741, "-", w740, ".tdms") -> (w732:string)
                                n521 = Create Folder(path (use dialog)=w746) -> (error out=w745:errorcluster)  [unwired: 2 in, 2 out]
                                n522 = call <vilib>:"Clear Errors.vi"("error in (no error)"=w745) -> ()  [unwired: 6 in, 1 out]
                                n523 = global write "Global 1.vi" "LAB01-1 FILE"(w732) -> ()
                              }
                              frame #1 {
                                (unwired) FALSE
                                n524 = String To Path(string=w753) -> (path=w751:path)
                                n525 = TDMS Open(6:FALSE, 10:T20."create or replace" ("operation (0:open)"), 11:w751) -> (0:w754:errorcluster, 3:→"TDMS LAB01-1":refnum<k34>)  [unwired: 4 in]
                              }
                              frame #2 {
                                n526 = local read "TDMS LAB01-1"() -> (w773:refnum<k34>)
                                n527 = local read "SET LAB01-1"() -> (w762:T5)
                                n528 = Build Array("Testers Name", "Description", "Set Test Cycles", "T-Rise minutes", "T-Rise Deg C") -> (w763:string[])
                                n529 = Unbundle(w762) -> ("NAME"=w761:string, "DESCRIPTION"=w760:string, "CYCLES"=w759:dbl, "T-RISE mins"=w758:dbl, "T-RISE deg C"=w757:dbl)
                                n530 = Number To Decimal String(number=w759) -> (decimal integer string=w772:string)  [unwired: 1 in]
                                n531 = Number To Decimal String(number=w758) -> (decimal integer string=w771:string)  [unwired: 1 in]
                                n532 = Number To Decimal String(number=w757) -> (decimal integer string=w770:string)  [unwired: 1 in]
                                n533 = Build Array(w761, w760, w772, w771, w770) -> (w769:string[])
                                n534 = TDMS Set Properties(5:w769, 7:w763, 11:w773) -> ()  [unwired: 3 in, 4 out]
                              }
                              frame #3 {
                                n535 = local read "DISP LAB01-1"() -> (w783:T4)
                                n536 = Concatenate Strings("LAB01-1  ", w775) -> (w774:string)
                                n537 = Two Button Dialog(message=w774, 1:w784, 2:w785) -> (T button?=w777:bool)
                                n538 = case shown="True" w777 {
                                tunnel: w783 -> [w788 w789]
                                tunnel: [w788 w789] -> w782
                                tunnel: [w787 w790] -> w781
                                tunnel: [w786 w790] -> w780
                                frame False {
                                n539 = Unbundle(w788) -> ("CYCLE"=w787:dbl, "MINS"=w786:dbl)  [unwired: 1 out]
                                }
                                frame True {
                                w790 = 0.0
                                }
                                }
                                n540 = Bundle(cluster=w782, "CYCLE"=w781, "MINS"=w780, "STATUS"="RUN") -> (w779:T4)
                                n541 = local write "DISP LAB01-1"(w779) -> ()
                              }
                              frame #4 {
                                n542 = local read "TEMP START LAB01-1"() -> (w793:cluster{"TL":dbl, "TN":dbl})
                                n543 = Bundle(cluster=w793, "TL"=w791, "TN"=w791) -> (w792:cluster{"TL":dbl, "TN":dbl})
                                n544 = local write "TEMP START LAB01-1"(w792) -> ()
                              }
                            }
                          }
                        }
                      }
                    }
                  }
                }
              }
              event "RUN LAB01-2": Value Change {
                n545 = event-data() -> ("NewVal"=w798:bool)  [unwired: 1 in, 5 out]
                n546 = local write "run lab01-2"(w798) -> ()
                n547 = case shown="True" w798 {
                  tunnel: w804 -> [_ w842]
                  tunnel: w803 -> [_ w841]
                  tunnel: w801 -> [w806 w840]
                  tunnel: w802 -> [_ w839]
                  tunnel: w800 -> [_ w838]
                  tunnel: [w805 w837] -> w799
                  tunnel: w797 -> [_ w836]
                  tunnel: w796 -> [_ w835]
                  tunnel: w795 -> [_ w834]
                  tunnel: w794 -> [_ w832]
                  frame False {
                    # "stop test"
                    n548 = stacked-sequence {
                      tunnel: w806 -> [w815 _]
                      tunnel: [w807 _] -> w805
                      frame #0 {
                        n549 = local read "DISP LAB01-2"() -> (w814:T4)
                        n550 = Unbundle(w814) -> ("CYCLE"=w812:dbl, "MINS"=w813:dbl)  [unwired: 1 out]
                        n551 = case shown="\"CHART TEST\", Default" w815 {
                          tunnel: w813 -> [_ _ w822]
                          tunnel: w812 -> [w820 w821 _]
                          tunnel: [w820 w821 w822] -> w811
                          frame "CHART TEST", Default {
                          }
                          frame "CYCLE TEST" {
                          }
                          frame "T-RISE TEST" {
                          }
                        }
                        n552 = local read "TDMS LAB01-2"() -> (w819:refnum<k34>)
                        n553 = Build Array("STOPPED") -> (w816:string[])
                        n554 = Build Array(w811) -> (w810:dbl[])
                        n555 = TDMS Write(0:w819, 5:"TEST RESULT", 7:w816, 9:w810) -> (4:w808:refnum<k34>, 15:w809:errorcluster)  [unwired: 2 in, 2 out]
                        n556 = TDMS Close(8:w809, 11:w808) -> (0:w807:errorcluster)  [unwired: 1 out]
                      }
                      frame #1 {
                        n557 = local read "DISP LAB01-2"() -> (w826:T4)
                        n558 = stacked-sequence {
                          tunnel: "LAB01-2" -> [w828 w830]
                          frame #0 {
                            n559 = call "sub vi - defrag tdms v1.vi"("panel id"=w828) -> ("error out"=w827:errorcluster)  [unwired: 10 in]
                            n560 = local write "data file error"(w827) -> ()
                          }
                          frame #1 {
                            n561 = call "Save data file (stop) v3.vi"("panel id"=w830) -> ("network file save error"=w829:errorcluster)  [unwired: 9 in, 1 out]
                            n562 = local write "RESULT LAB01-2"(FALSE) -> ()
                            n563 = local write "data file error"(w829) -> ()
                          }
                        }
                        n564 = Bundle(cluster=w826, "STATUS"="STOP") -> (w824:T4)  [unwired: 2 in]
                        n565 = local write "DISP LAB01-2"(w824) -> ()
                      }
                    }
                  }
                  frame True {
                    n566 = local read "SIG LAB01-2"() -> (w833:T2)
                    n567 = stacked-sequence {
                      seq-local: [w844 _] -> [_ w848]
                      tunnel: w842 -> [_ w858]
                      tunnel: w841 -> [_ w857]
                      tunnel: w840 -> [_ w856]
                      tunnel: w839 -> [_ w855]
                      tunnel: w838 -> [_ w854]
                      tunnel: [_ w853] -> w837
